vi "Config Dev Auto.vi"(8 "error in":errorcluster, 9 "Loss (off)":bool, 10 "Capacitance (off)":bool, 11 "VISA resource name":refnum<visa-resource-name>) -> (0 "error out":errorcluster, 3 "VISA resource name out":refnum<visa-resource-name>)   [LabVIEW 2017, in "Andeen-Hagerling 2700.lvlib"]
doc: "During each initialization of the deviation mode the DUT is measured resulting in a set of capacitance and loss values known as the Initial Deviation Reading. These values may be used to automatically establish new Deviation Setpoint values. Alternatively, the Deviation Setpoints remain fixed at their previous values and the Initial Deviation Readings are used simply to verify that the DUT is within the previously\nspecified upper and lower boundaries."
uses:
  Andeen-Hagerling 2700.lvlib
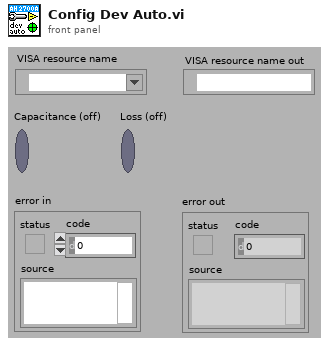
[diagram p1: front panel]
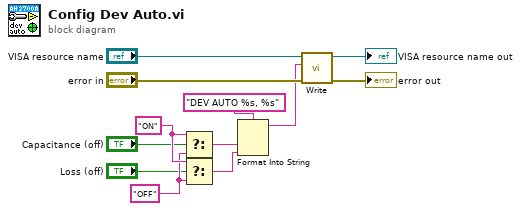
[diagram p0: block diagram]
diagram:
  w7 = "OFF"
  w8 = "ON"
  n1 = Select(t=w8, s="Capacitance (off)", f=w7) -> (s? t:f=w2:string)
  n2 = Select(t=w8, s="Loss (off)", f=w7) -> (s? t:f=w1:string)
  n3 = Format Into String(format string="DEV AUTO %s, %s", w2, w1) -> (resulting string=w3:string)  [unwired: 2 in, 1 out]
  n4 = call "Write.vi"("error in"="error in", "command"=w3, "VISA resource name"="VISA resource name") -> ("error out"=→"error out":errorcluster, "VISA resource name out"=→"VISA resource name out":refnum<visa-resource-name>)  [unwired: 7 in]
